vi "REACTOR__SET_TIME_CONSTANT_TEMP.vi"(6 "error in (no error)":errorcluster, 7 "Index":i8) -> (0 "error out":errorcluster, 2 "resulting string 1":string="Mide Bronkhorst 1, mide Alicats 1,  y pausa 1.0s", 3 "Cancelled?":bool)   [LabVIEW 2017]
doc: "Use this template to create a dialog box. This template polls the state of the buttons on the front panel and does not use events. Use the Dialog Using Events template (not available in Base package) to create a dialog box with event handling."
panel:
  in  "Tiempo (min)":dbl=5.0
  in  "Pausa (s)":dbl=5.0
  in  "Cancel":bool
  in  "OK":bool
  # "MANTENER \nTEMPERATURA CONSTANTE"
  # "Asegurese de que se han indicado \nlos parámetros a medir"
  # "Noviembre 2022 V1.0  a-sslcdms"
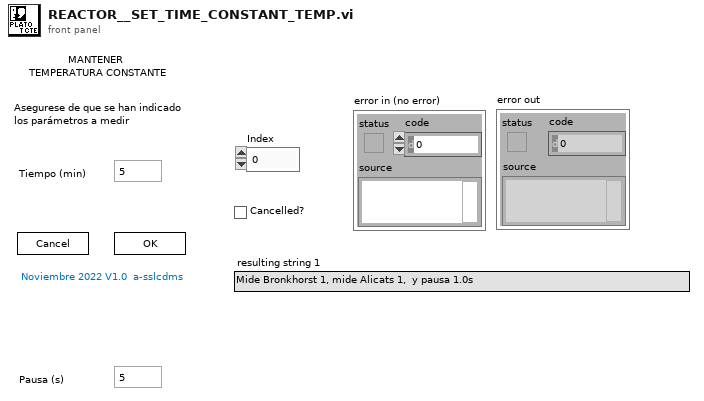
[diagram p1: front panel]
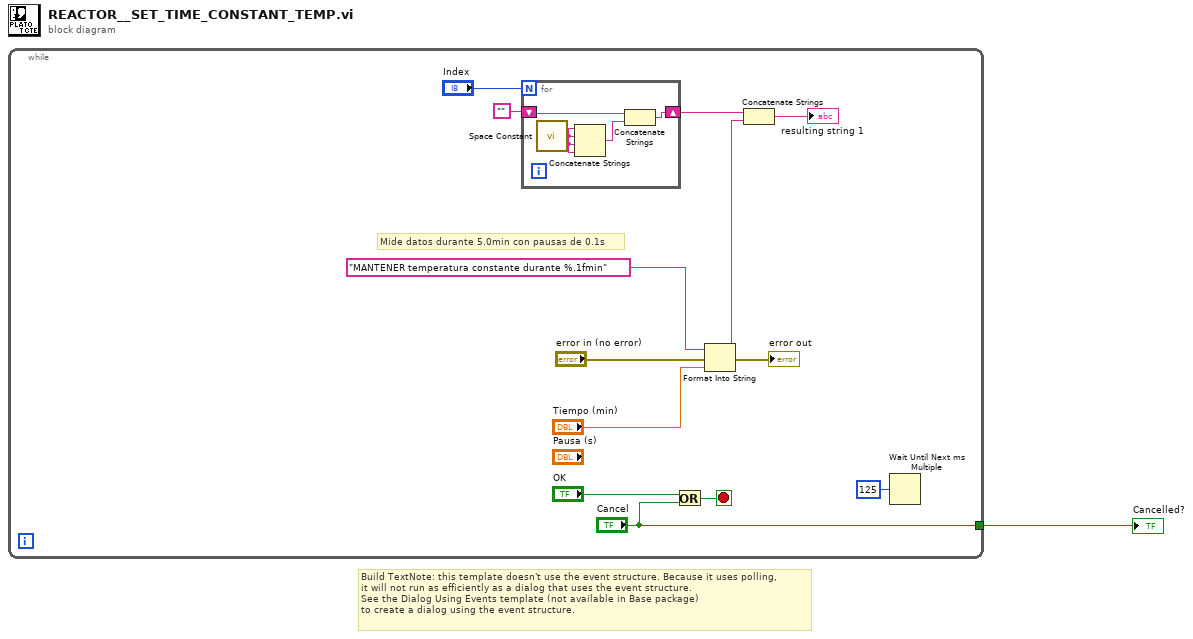
[diagram p0: block diagram]
diagram:
  # "Build TextNote: this template doesn't use the event structure. Because it uses polling, \nit will not run as efficiently as a dialog that uses the event structure.\nSee the Dialog Using Events template (not available in Base package) \nto create a dialog using the event structure."
  n1 = while {
    tunnel: ["Cancel"] -> w1
    stop <- w13 stop-if-true
    # "Mide datos durante 5.0min con pausas de 0.1s"
    n2 = for {
      N: "Index" -> [_]
      shift-right: [w17] -> w5
      shift-left: "" -> [w16]
      n3 = call <vilib>:"Space Constant.vi"() -> ("String"=w15:string)
      n4 = Concatenate Strings(w15, w15, w15, w15) -> (w18:string)
      n5 = Concatenate Strings(w16, w18) -> (w17:string)
    }
    n6 = Or(x="OK", y="Cancel") -> (x .or. y?=w13:bool)
    n7 = Format Into String(format string="MANTENER temperatura constante durante %.1fmin", error in="error in (no error)", "Tiempo (min)") -> (resulting string=w3:string, error out=→"error out":errorcluster)  [unwired: 1 in]
    n8 = Concatenate Strings(w5, w3) -> (→"resulting string 1":string)
    n9 = Wait Until Next ms Multiple(millisecond multiple=u32 125) -> ()  [unwired: 1 out]
  }
  "Cancelled?" <- w1
